vi "1_01.vi"() -> ()   [LabVIEW 2013]
panel:
  out "String":string
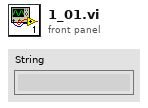
[diagram p1: front panel]
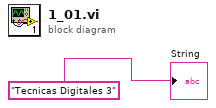
[diagram p0: block diagram]
diagram:
  "String" <- "Tecnicas Digitales 3"
